vi "Destroy.vi"(8 "ErrorIn":errorcluster caption="Error In(no Error)", 11 "Reference in":refnum<class "ErrorDefinitionSQLite.lvclass"> caption="Reference In") -> (0 "ErrorOut":errorcluster caption="Error Out", 3 "Reference out":refnum<class "ErrorDefinitionSQLite.lvclass"> caption="Reference Out")   [LabVIEW 2018, in "ErrorDefinitionSQLite.lvclass"]
uses:
  <userlib>/_express/CustomErrorCreator/ErrorDefinitionSQLite/ErrorDefinitionSQLite.lvclass
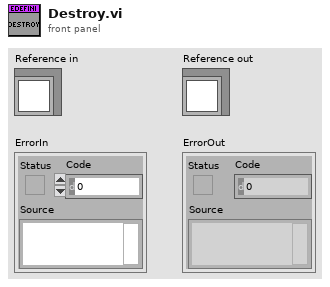
[diagram p1: front panel]
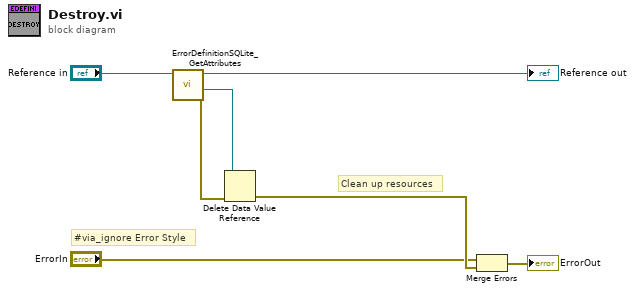
[diagram p0: block diagram]
diagram:
  # "#via_ignore Error Style"
  # "Clean up resources"
  n1 = call <userlib>:"ErrorDefinitionSQLite_GetAttributes.vi"("Reference in"="Reference in") -> ("ErrorOut"=w4:errorcluster, "DataRef"=w3:refnum<data-value>, "Reference out"=→"Reference out":refnum<class "ErrorDefinitionSQLite.lvclass">)  [unwired: 7 in, 1 out]
  n2 = Delete Data Value Reference(data value reference=w3, error in=w4) -> (error out=w2:errorcluster)  [unwired: 1 out]
  n3 = Merge Errors("ErrorIn", w2) -> (→"ErrorOut":errorcluster)
